vi "水样测试.vi"(11 "数据标记表":string(combo)="N") -> ()   [LabVIEW 2016, in "斯坦道多参数.lvlib"]
panel:
  out "运行状态":u16(ring) items=["空闲", "水样测试", "标样核查"]
  out "多参数运行日志":string
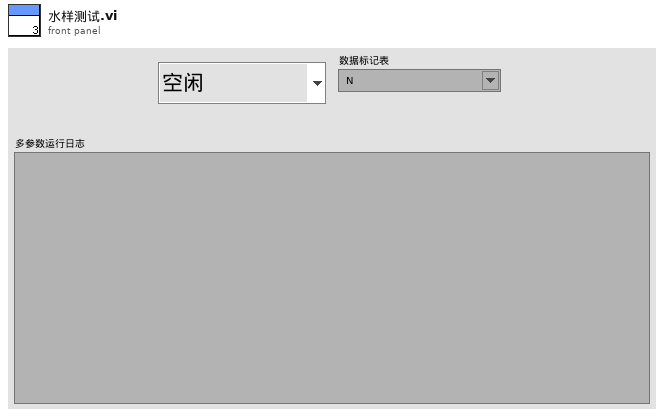
[diagram p1: front panel]
types:
  T1 = cluster{"水样数据时间":timestamp, "水温":dbl, "pH":dbl, "DO":dbl, "DOper":dbl, "电导率":dbl, "ORP":dbl, "浊度":dbl, "叶绿素a":dbl, "藻密度":dbl}
  T2 = cluster{"水温":bool, "pH":bool, "DO":bool, "DOper":bool, "电导率":bool, "ORP":bool, "浊度":bool, "叶绿素a":bool, "藻密度":bool}
  T3 = cluster{"水样数据时间":timestamp, "测量模式":string, "数据类型":string, "水样实测值":sgl, "单位":string, "水样数据标识":string, "信号值":sgl, "标样参考值":sgl, "因子编码":string, "探头温度":sgl}
  T4 = cluster{"ph":bool, "DO":bool, "Cond":bool, "Turb":bool, "叶绿素a":bool, "藻密度":bool, "ORP":bool}
  T5 = cluster{"CH":u16, "监测值":dbl, "温度偏移修正值":sgl, "信号值":sgl}
  T6 = cluster{"温度测量值":sgl, "测量值":sgl, "温度偏移修正值":sgl, "信号值":sgl}
  T7 = cluster{"温度测量值":sgl, "DO%":sgl, "DOmg/L":sgl, "温度偏移修正值":sgl}
  T8 = cluster{"测量量程":dbl, "测量精度":dbl, "测量间隔":dbl, "消解温度":dbl, "消解时长":dbl, "空白校准时间":timestamp, "曲线截距":dbl, "曲线斜率":dbl, "测量检出限":dbl, "测量信号值":dbl, "线性相关系数":dbl, "二次多项式系数":dbl, "标样校准时间":timestamp, "稀释倍数":dbl, "三项式系数":dbl, "空白标定系数":dbl, "量程系数":dbl, "F0/ORPA":dbl, "F1/ORPB":dbl, "F2/ORPK":dbl, "F3":dbl, "F4":dbl, "F5":dbl, "F6":dbl, "F7":dbl, "X0/滴定数":dbl, "量程":dbl}
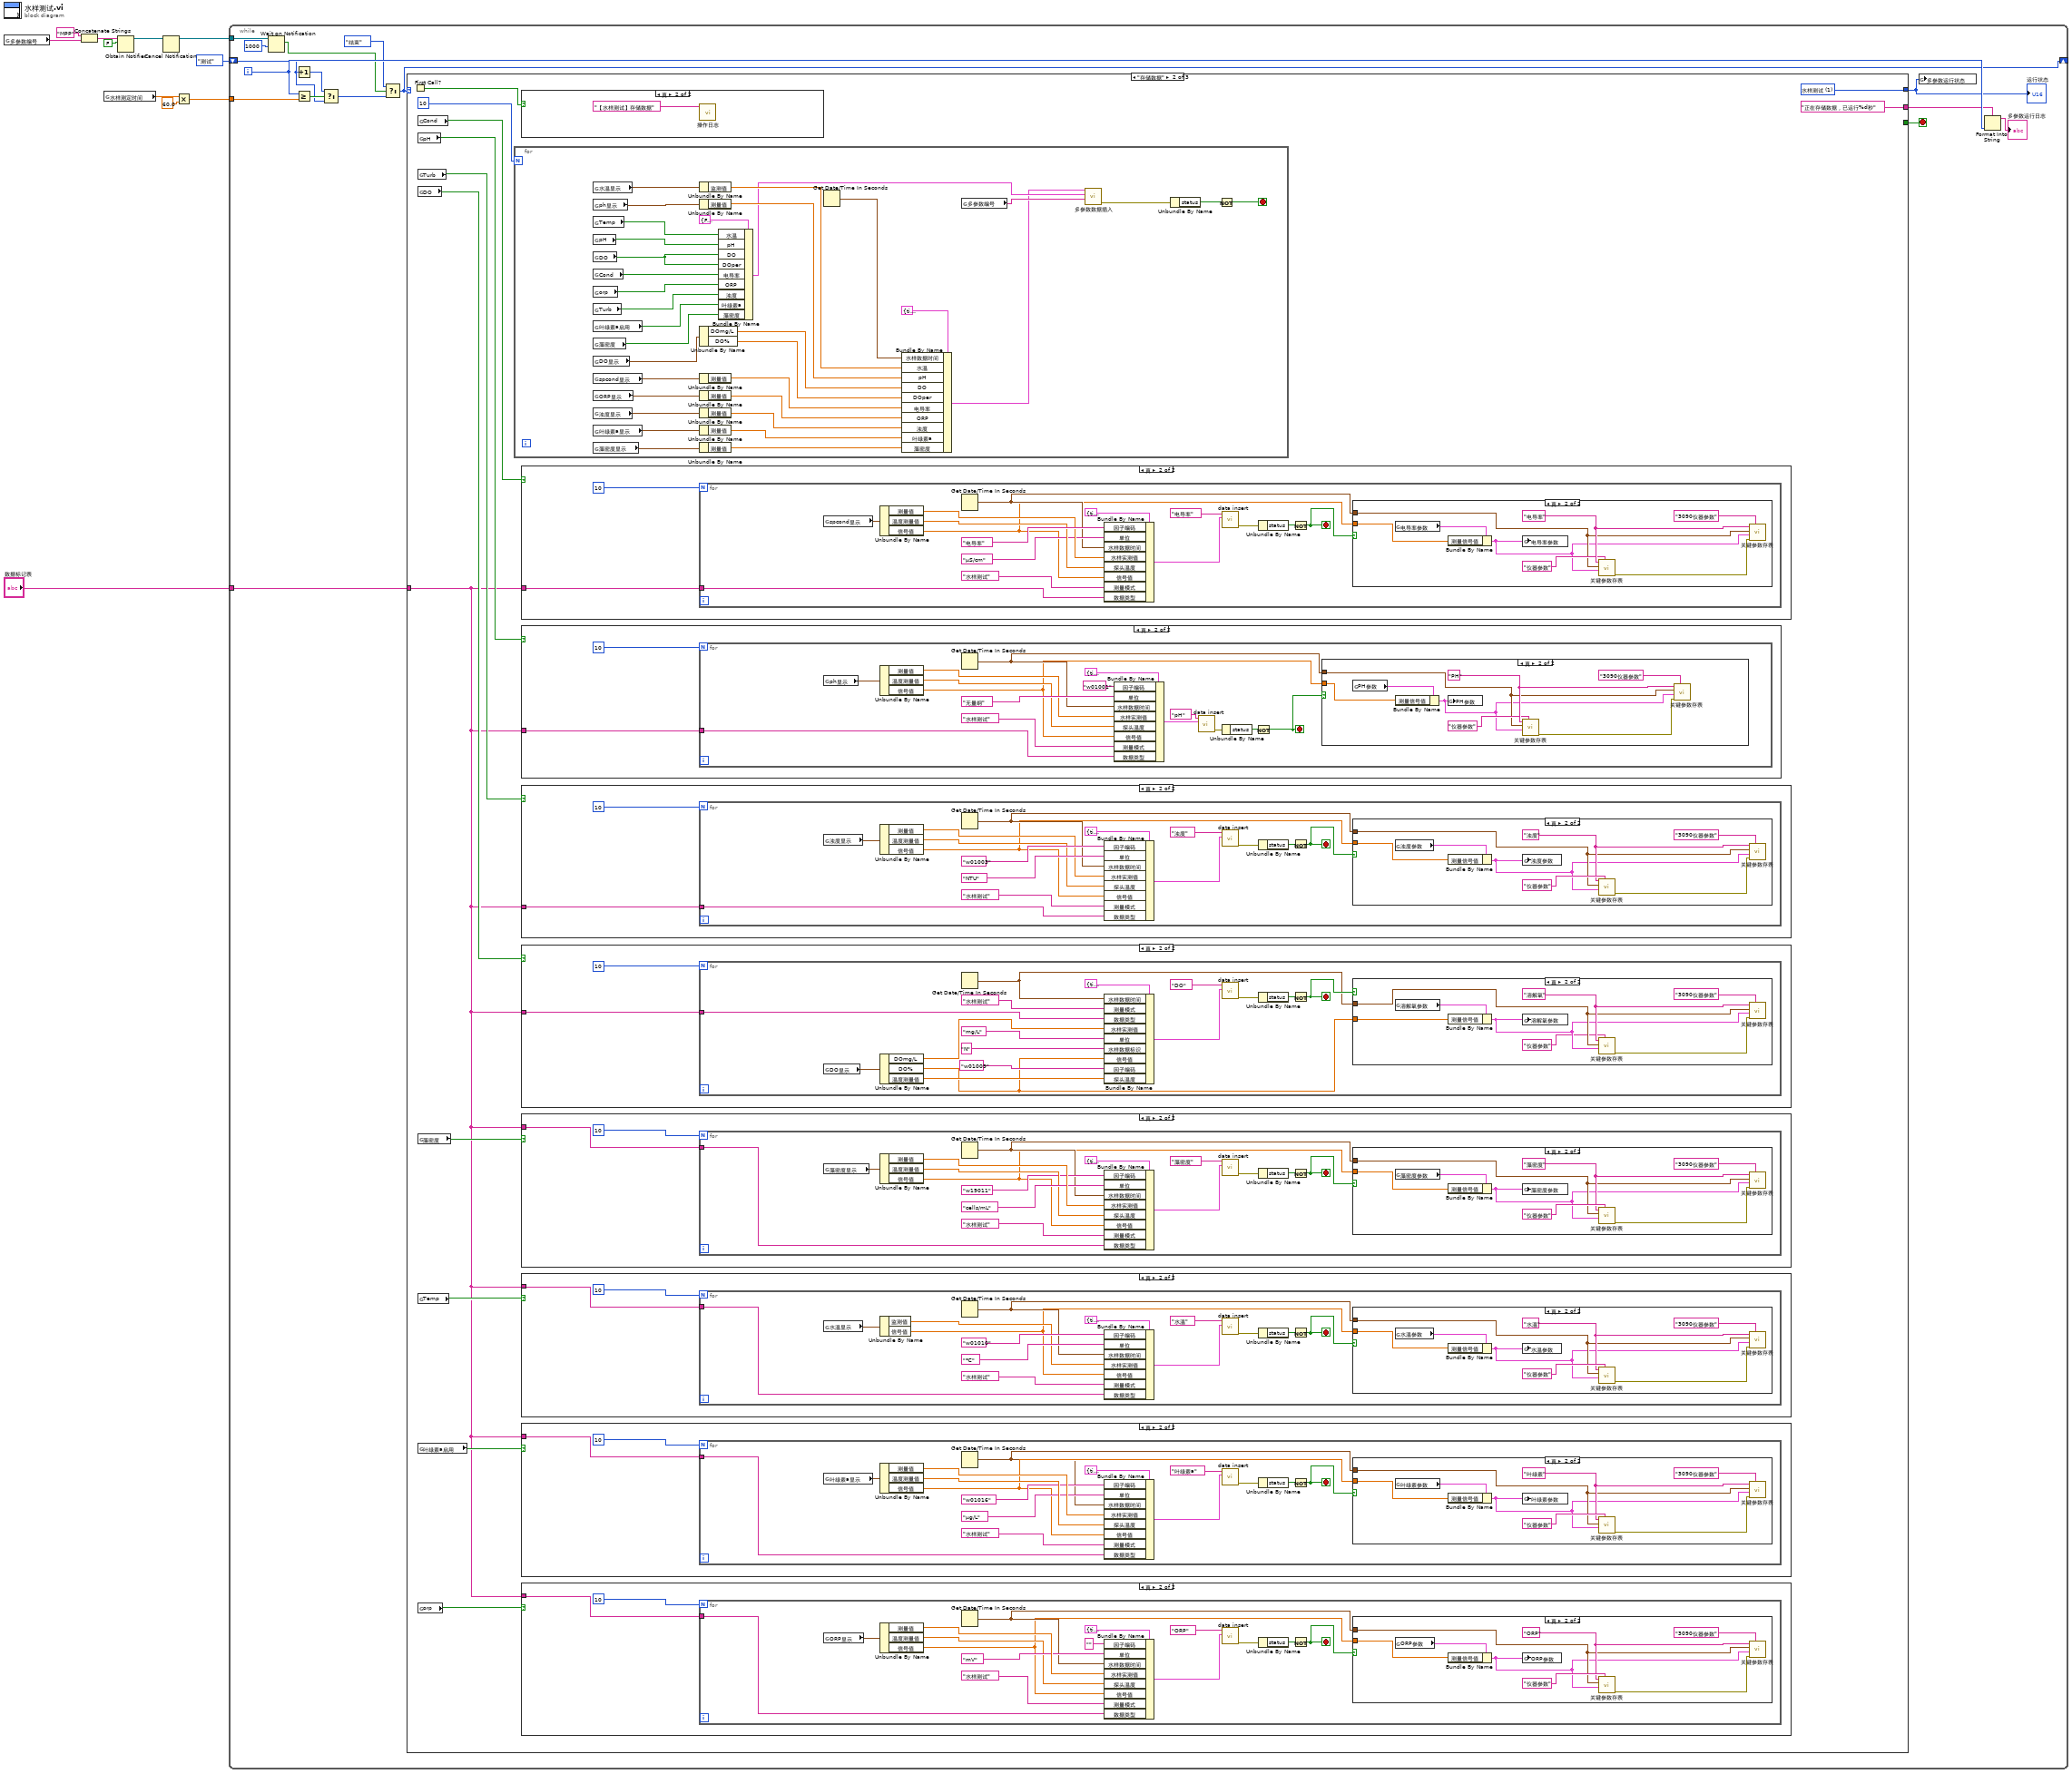
[diagram p0: block diagram]
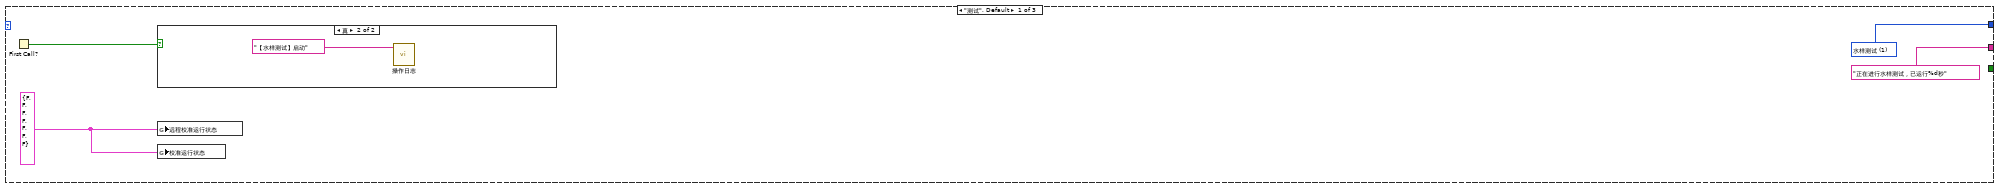
[diagram p2: hidden frame]
diagram:
  n1 = global read "多参数全局变量.vi" "多参数编号"() -> (w2:string)
  n2 = Concatenate Strings("MPP" ("名称（未命名）"), w2) -> (w3:string)
  n3 = global read "断电保存变量.vi" "水样测定时间"() -> (w1:dbl)
  n4 = Obtain Notifier(name (unnamed)=w3, notification data type=FALSE) -> (notifier out=w6:refnum<notifier>)  [unwired: 2 in, 2 out]
  n5 = Cancel Notification(0:w6) -> (8:w5:refnum<notifier>)  [unwired: 1 in, 2 out]
  n6 = Multiply(x=w1, y=60.0) -> (x*y=w10:dbl)
  n7 = while {
    tunnel: w10 -> [w27]
    shift-right: [w14] -> _
    shift-left: enum16{"测试", "存储数据", "结束"}."测试" ("枚举") -> [w21]
    tunnel: w5 -> [w19]
    tunnel: "数据标记表" -> [w13]
    i -> [w25]
    stop <- w26 stop-if-true
    n8 = Wait on Notification(notifier=w19, timeout in ms (-1)=1000 ("超时毫秒(-1)")) -> (notification=w17:bool)  [unwired: 2 in, 3 out]
    n9 = Increment(x=w21) -> (x+1=w20:enum16{"测试", "存储数据", "结束"})
    n10 = Greater Or Equal?(x=w25, y=w27) -> (x >= y?=w22:bool)
    n11 = Select(t=w20, s=w22, f=w21) -> (s? t:f=w15:enum16{"测试", "存储数据", "结束"})
    n12 = Select(t=enum16{"测试", "存储数据", "结束"}."结束" ("枚举"), s=w17, f=w15) -> (s? t:f=w14:enum16{"测试", "存储数据", "结束"})
    n13 = case shown="\"存储数据\"" w14 {
      tunnel: [_ _ TRUE] -> w26
      tunnel: ["正在进行水样测试，已运行%d秒" ("格式字符串") "正在存储数据，已运行%d秒" ("格式字符串") "测试停止，累计运行%d秒" ("格式字符串")] -> w24
      tunnel: [w30 w38 w282] -> w12
      tunnel: w13 -> [_ w35 _]
      frame "测试", Default {
        w28 = T4 {"ph"=FALSE, "DO"=FALSE, "Cond"=FALSE, "Turb"=FALSE, "叶绿素a"=FALSE, "藻密度"=FALSE, "ORP"=FALSE} ("校准运行状态")
        w30 = u16 1 items=["空闲", "水样测试", "标样核查"] ("多参数运行状态")
        n14 = First Call?() -> (First Call?: T/F=w29:bool)
        n15 = case shown="真" w29 {
          frame False {
          }
          frame True {
            n16 = call "操作日志.vi"("日志信息"="【水样测试】启动") -> ()  [unwired: 10 in, 1 out]
          }
        }
        n17 = global write "多参数全局变量.vi" "远程校准运行状态"(w28) -> ()
        n18 = global write "多参数全局变量.vi" "校准运行状态"(w28) -> ()
      }
      frame "存储数据" {
        w38 = u16 1 items=["空闲", "水样测试", "标样核查"] ("多参数运行状态")
        n19 = First Call?() -> (First Call?: T/F=w36:bool)
        n20 = global read "断电保存变量.vi" "Cond"() -> (w43:bool)
        n21 = global read "断电保存变量.vi" "pH"() -> (w41:bool)
        n22 = global read "断电保存变量.vi" "Turb"() -> (w44:bool)
        n23 = global read "断电保存变量.vi" "DO"() -> (w42:bool)
        n24 = global read "断电保存变量.vi" "藻密度"() -> (w37:bool)
        n25 = global read "断电保存变量.vi" "Temp"() -> (w40:bool)
        n26 = global read "断电保存变量.vi" "叶绿素a启用"() -> (w45:bool)
        n27 = global read "断电保存变量.vi" "orp"() -> (w34:bool)
        n28 = for {
          N: 10 -> [_]
          stop <- w49 stop-if-true
          n29 = global read "多参数全局变量.vi" "水温显示"() -> (w78:T5)
          n30 = global read "多参数全局变量.vi" "ph显示"() -> (w76:T6)
          n31 = global read "断电保存变量.vi" "Temp"() -> (w56:bool)
          n32 = global read "断电保存变量.vi" "pH"() -> (w60:bool)
          n33 = global read "断电保存变量.vi" "DO"() -> (w52:bool)
          n34 = global read "断电保存变量.vi" "Cond"() -> (w59:bool)
          n35 = global read "断电保存变量.vi" "orp"() -> (w55:bool)
          n36 = global read "断电保存变量.vi" "Turb"() -> (w58:bool)
          n37 = global read "断电保存变量.vi" "叶绿素a启用"() -> (w54:bool)
          n38 = global read "断电保存变量.vi" "藻密度"() -> (w57:bool)
          n39 = global read "多参数全局变量.vi" "DO显示"() -> (w74:T7)
          n40 = global read "多参数全局变量.vi" "spcond显示"() -> (w71:T6)
          n41 = global read "多参数全局变量.vi" "ORP显示"() -> (w69:T6)
          n42 = global read "多参数全局变量.vi" "浊度显示"() -> (w67:T6)
          n43 = global read "多参数全局变量.vi" "叶绿素a显示"() -> (w63:T6)
          n44 = global read "多参数全局变量.vi" "藻密度显示"() -> (w65:T6)
          n45 = Unbundle By Name(w78) -> ("监测值"=w77:dbl)
          n46 = Unbundle By Name(w76) -> ("测量值"=w75:sgl)
          n47 = Unbundle By Name(w74) -> ("DOmg/L"=w73:sgl, "DO%"=w72:sgl)
          n48 = Unbundle By Name(w71) -> ("测量值"=w70:sgl)
          n49 = Unbundle By Name(w69) -> ("测量值"=w68:sgl)
          n50 = Unbundle By Name(w67) -> ("测量值"=w66:sgl)
          n51 = Unbundle By Name(w63) -> ("测量值"=w62:sgl)
          n52 = Unbundle By Name(w65) -> ("测量值"=w64:sgl)
          n53 = Bundle By Name(cluster=T2 {"水温"=FALSE, "pH"=FALSE, "DO"=FALSE, "DOper"=FALSE, "电导率"=FALSE, "ORP"=FALSE, "浊度"=FALSE, "叶绿素a"=FALSE, "藻密度"=FALSE} ("columns enable"), "水温"=w56, "pH"=w60, "DO"=w52, "DOper"=w52, "电导率"=w59, "ORP"=w55, "浊度"=w58, "叶绿素a"=w54, "藻密度"=w57) -> (w53:T2)
          n54 = Get Date/Time In Seconds() -> (seconds since 1Jan1904=w79:timestamp)
          n55 = Bundle By Name(cluster=T1 {"水样数据时间"=timestamp(0 s since 1904-01-01), "水温"=0.0, "pH"=0.0, "DO"=0.0, "DOper"=0.0, "电导率"=0.0, "ORP"=0.0, "浊度"=0.0, "叶绿素a"=0.0, "藻密度"=0.0} ("data in"), "水样数据时间"=w79, "水温"=w77, "pH"=w75, "DO"=w73, "DOper"=w72, "电导率"=w70, "ORP"=w68, "浊度"=w66, "叶绿素a"=w62, "藻密度"=w64) -> (w46:T1)
          n56 = global read "多参数全局变量.vi" "多参数编号"() -> (w48:string)
          n57 = call "多参数数据插入.vi"("编号"=w48, "columns enable"=w53, "data in"=w46) -> ("error out"=w51:errorcluster)  [unwired: 8 in]
          n58 = Unbundle By Name(w51) -> ("status"=w50:bool)
          n59 = Not(x=w50) -> (.not. x?=w49:bool)
        }
        n60 = case shown="真" w36 {
          frame False {
          }
          frame True {
            n61 = call "操作日志.vi"("日志信息"="【水样测试】存储数据") -> ()  [unwired: 10 in, 1 out]
          }
        }
        n62 = case shown="真" w43 {
          tunnel: w35 -> [_ w182]
          frame False {
          }
          frame True {
            n63 = for {
              N: 10 -> [_]
              tunnel: w182 -> [w183]
              stop <- w189 stop-if-true
              n64 = global read "多参数全局变量.vi" "spcond显示"() -> (w195:T6)
              n65 = Unbundle By Name(w195) -> ("测量值"=w194:sgl, "温度测量值"=w193:sgl, "信号值"=w187:sgl)
              n66 = Get Date/Time In Seconds() -> (seconds since 1Jan1904=w188:timestamp)
              n67 = Bundle By Name(cluster=T3 {"水样数据时间"=timestamp(0 s since 1904-01-01), "测量模式"="", "数据类型"="N", "水样实测值"=0.0, "单位"="", "水样数据标识"="N", "信号值"=0.0, "标样参考值"=0.0, "因子编码"="", "探头温度"=0.0} ("data in"), "因子编码"="电导率", "单位"="μS/cm", "水样数据时间"=w188, "水样实测值"=w194, "探头温度"=w193, "信号值"=w187, "测量模式"="水样测试", "数据类型"=w183) -> (w184:T3)
              n68 = call "data insert.vi"("data in"=w184, "table in"="电导率" ("table输入")) -> ("error out"=w192:errorcluster)  [unwired: 9 in]
              n69 = Unbundle By Name(w192) -> ("status"=w191:bool)
              n70 = Not(x=w191) -> (.not. x?=w189:bool)
              n71 = case shown="真" w189 {
                tunnel: w188 -> [_ w200]
                tunnel: w187 -> [_ w204]
                frame False {
                }
                frame True {
                  w203 = "电导率" ("仪器名称")
                  n72 = global read "断电保存变量.vi" "电导率参数"() -> (w205:T8)
                  n73 = Bundle By Name(cluster=w205, "测量信号值"=w204) -> (w199:T8)
                  n74 = global write "断电保存变量.vi" "电导率参数"(w199) -> ()
                  n75 = call "关键参数存表.vi"("table"="仪器参数", "仪器参数"=w199, "datatime"=w200, "仪器名称"=w203) -> ("error out"=w198:errorcluster)  [unwired: 7 in]
                  n76 = call "关键参数存表.vi"("table"="3090仪器参数", "error in (no error)"=w198, "仪器参数"=w199, "datatime"=w200, "仪器名称"=w203) -> ()  [unwired: 6 in, 1 out]
                }
              }
            }
          }
        }
        n77 = case shown="真" w41 {
          tunnel: w35 -> [_ w233]
          frame False {
          }
          frame True {
            n78 = for {
              N: 10 -> [_]
              tunnel: w233 -> [w234]
              stop <- w239 stop-if-true
              n79 = global read "多参数全局变量.vi" "ph显示"() -> (w244:T6)
              n80 = Unbundle By Name(w244) -> ("测量值"=w243:sgl, "温度测量值"=w242:sgl, "信号值"=w237:sgl)
              n81 = Get Date/Time In Seconds() -> (seconds since 1Jan1904=w238:timestamp)
              n82 = Bundle By Name(cluster=T3 {"水样数据时间"=timestamp(0 s since 1904-01-01), "测量模式"="", "数据类型"="N", "水样实测值"=0.0, "单位"="", "水样数据标识"="N", "信号值"=0.0, "标样参考值"=0.0, "因子编码"="", "探头温度"=0.0} ("data in"), "因子编码"="w01001", "单位"="无量纲", "水样数据时间"=w238, "水样实测值"=w243, "探头温度"=w242, "信号值"=w237, "测量模式"="水样测试", "数据类型"=w234) -> (w248:T3)
              n83 = call "data insert.vi"("data in"=w248, "table in"="pH" ("table输入")) -> ("error out"=w241:errorcluster)  [unwired: 9 in]
              n84 = Unbundle By Name(w241) -> ("status"=w240:bool)
              n85 = Not(x=w240) -> (.not. x?=w239:bool)
              n86 = case shown="真" w239 {
                tunnel: w238 -> [_ w251]
                tunnel: w237 -> [_ w255]
                frame False {
                }
                frame True {
                  w254 = "PH" ("仪器名称")
                  n87 = global read "断电保存变量.vi" "PH参数"() -> (w256:T8)
                  n88 = Bundle By Name(cluster=w256, "测量信号值"=w255) -> (w250:T8)
                  n89 = global write "断电保存变量.vi" "PH参数"(w250) -> ()
                  n90 = call "关键参数存表.vi"("table"="仪器参数", "仪器参数"=w250, "datatime"=w251, "仪器名称"=w254) -> ("error out"=w249:errorcluster)  [unwired: 7 in]
                  n91 = call "关键参数存表.vi"("table"="3090仪器参数", "error in (no error)"=w249, "仪器参数"=w250, "datatime"=w251, "仪器名称"=w254) -> ()  [unwired: 6 in, 1 out]
                }
              }
            }
          }
        }
        n92 = case shown="真" w44 {
          tunnel: w35 -> [_ w157]
          frame False {
          }
          frame True {
            n93 = for {
              N: 10 -> [_]
              tunnel: w157 -> [w158]
              stop <- w163 stop-if-true
              n94 = global read "多参数全局变量.vi" "浊度显示"() -> (w168:T6)
              n95 = Unbundle By Name(w168) -> ("测量值"=w167:sgl, "温度测量值"=w166:sgl, "信号值"=w161:sgl)
              n96 = Get Date/Time In Seconds() -> (seconds since 1Jan1904=w162:timestamp)
              n97 = Bundle By Name(cluster=T3 {"水样数据时间"=timestamp(0 s since 1904-01-01), "测量模式"="", "数据类型"="N", "水样实测值"=0.0, "单位"="", "水样数据标识"="N", "信号值"=0.0, "标样参考值"=0.0, "因子编码"="", "探头温度"=0.0} ("data in"), "因子编码"="w01003", "单位"="NTU", "水样数据时间"=w162, "水样实测值"=w167, "探头温度"=w166, "信号值"=w161, "测量模式"="水样测试", "数据类型"=w158) -> (w171:T3)
              n98 = call "data insert.vi"("data in"=w171, "table in"="浊度" ("table输入")) -> ("error out"=w165:errorcluster)  [unwired: 9 in]
              n99 = Unbundle By Name(w165) -> ("status"=w164:bool)
              n100 = Not(x=w164) -> (.not. x?=w163:bool)
              n101 = case shown="真" w163 {
                tunnel: w162 -> [_ w175]
                tunnel: w161 -> [_ w179]
                frame False {
                }
                frame True {
                  w176 = "浊度" ("仪器名称")
                  n102 = global read "断电保存变量.vi" "浊度参数"() -> (w180:T8)
                  n103 = Bundle By Name(cluster=w180, "测量信号值"=w179) -> (w174:T8)
                  n104 = global write "断电保存变量.vi" "浊度参数"(w174) -> ()
                  n105 = call "关键参数存表.vi"("table"="仪器参数", "仪器参数"=w174, "datatime"=w175, "仪器名称"=w176) -> ("error out"=w173:errorcluster)  [unwired: 7 in]
                  n106 = call "关键参数存表.vi"("table"="3090仪器参数", "error in (no error)"=w173, "仪器参数"=w174, "datatime"=w175, "仪器名称"=w176) -> ()  [unwired: 6 in, 1 out]
                }
              }
            }
          }
        }
        n107 = case shown="真" w42 {
          tunnel: w35 -> [_ w207]
          frame False {
          }
          frame True {
            n108 = for {
              N: 10 -> [_]
              tunnel: w207 -> [w218]
              stop <- w222 stop-if-true
              n109 = global read "多参数全局变量.vi" "DO显示"() -> (w223:T7)
              n110 = Unbundle By Name(w223) -> ("DOmg/L"=w217:sgl, "DO%"=w210:sgl, "温度测量值"=w211:sgl)
              n111 = Get Date/Time In Seconds() -> (seconds since 1Jan1904=w220:timestamp)
              n112 = Bundle By Name(cluster=T3 {"水样数据时间"=timestamp(0 s since 1904-01-01), "测量模式"="", "数据类型"="N", "水样实测值"=0.0, "单位"="", "水样数据标识"="N", "信号值"=0.0, "标样参考值"=0.0, "因子编码"="", "探头温度"=0.0} ("data in"), "水样数据时间"=w220, "测量模式"="水样测试", "数据类型"=w218, "水样实测值"=w217, "单位"="mg/L", "水样数据标识"="N", "信号值"=w210, "因子编码"="w01009", "探头温度"=w211) -> (w208:T3)
              n113 = call "data insert.vi"("data in"=w208, "table in"="DO") -> ("error out"=w213:errorcluster)  [unwired: 9 in]
              n114 = Unbundle By Name(w213) -> ("status"=w214:bool)
              n115 = Not(x=w214) -> (.not. x?=w222:bool)
              n116 = case shown="真" w222 {
                tunnel: w220 -> [_ w228]
                tunnel: w210 -> [_ w230]
                frame False {
                }
                frame True {
                  w229 = "溶解氧" ("仪器名称")
                  n117 = global read "断电保存变量.vi" "溶解氧参数"() -> (w231:T8)
                  n118 = Bundle By Name(cluster=w231, "测量信号值"=w230) -> (w227:T8)
                  n119 = global write "断电保存变量.vi" "溶解氧参数"(w227) -> ()
                  n120 = call "关键参数存表.vi"("table"="仪器参数", "仪器参数"=w227, "datatime"=w228, "仪器名称"=w229) -> ("error out"=w226:errorcluster)  [unwired: 7 in]
                  n121 = call "关键参数存表.vi"("table"="3090仪器参数", "error in (no error)"=w226, "仪器参数"=w227, "datatime"=w228, "仪器名称"=w229) -> ()  [unwired: 6 in, 1 out]
                }
              }
            }
          }
        }
        n122 = case shown="真" w37 {
          tunnel: w35 -> [_ w107]
          frame False {
          }
          frame True {
            n123 = for {
              N: 10 -> [_]
              tunnel: w107 -> [w109]
              stop <- w111 stop-if-true
              n124 = global read "多参数全局变量.vi" "藻密度显示"() -> (w117:T6)
              n125 = Unbundle By Name(w117) -> ("测量值"=w122:sgl, "温度测量值"=w120:sgl, "信号值"=w112:sgl)
              n126 = Get Date/Time In Seconds() -> (seconds since 1Jan1904=w113:timestamp)
              n127 = Bundle By Name(cluster=T3 {"水样数据时间"=timestamp(0 s since 1904-01-01), "测量模式"="", "数据类型"="N", "水样实测值"=0.0, "单位"="", "水样数据标识"="N", "信号值"=0.0, "标样参考值"=0.0, "因子编码"="", "探头温度"=0.0} ("data in"), "因子编码"="w19011", "单位"="cells/mL", "水样数据时间"=w113, "水样实测值"=w122, "探头温度"=w120, "信号值"=w112, "测量模式"="水样测试", "数据类型"=w109) -> (w114:T3)
              n128 = call "data insert.vi"("data in"=w114, "table in"="藻密度" ("table输入")) -> ("error out"=w116:errorcluster)  [unwired: 9 in]
              n129 = Unbundle By Name(w116) -> ("status"=w115:bool)
              n130 = Not(x=w115) -> (.not. x?=w111:bool)
              n131 = case shown="真" w111 {
                tunnel: w113 -> [_ w126]
                tunnel: w112 -> [_ w129]
                frame False {
                }
                frame True {
                  w127 = "藻密度" ("仪器名称")
                  n132 = global read "断电保存变量.vi" "藻密度参数"() -> (w130:T8)
                  n133 = Bundle By Name(cluster=w130, "测量信号值"=w129) -> (w125:T8)
                  n134 = global write "断电保存变量.vi" "藻密度参数"(w125) -> ()
                  n135 = call "关键参数存表.vi"("table"="仪器参数", "仪器参数"=w125, "datatime"=w126, "仪器名称"=w127) -> ("error out"=w124:errorcluster)  [unwired: 7 in]
                  n136 = call "关键参数存表.vi"("table"="3090仪器参数", "error in (no error)"=w124, "仪器参数"=w125, "datatime"=w126, "仪器名称"=w127) -> ()  [unwired: 6 in, 1 out]
                }
              }
            }
          }
        }
        n137 = case shown="真" w40 {
          tunnel: w35 -> [_ w258]
          frame False {
          }
          frame True {
            n138 = for {
              N: 10 -> [_]
              tunnel: w258 -> [w259]
              stop <- w264 stop-if-true
              n139 = global read "多参数全局变量.vi" "水温显示"() -> (w268:T5)
              n140 = Unbundle By Name(w268) -> ("监测值"=w267:dbl, "信号值"=w262:sgl)
              n141 = Get Date/Time In Seconds() -> (seconds since 1Jan1904=w263:timestamp)
              n142 = Bundle By Name(cluster=T3 {"水样数据时间"=timestamp(0 s since 1904-01-01), "测量模式"="", "数据类型"="N", "水样实测值"=0.0, "单位"="", "水样数据标识"="N", "信号值"=0.0, "标样参考值"=0.0, "因子编码"="", "探头温度"=0.0} ("data in"), "因子编码"="w01010", "单位"="℃", "水样数据时间"=w263, "水样实测值"=w267, "信号值"=w262, "测量模式"="水样测试", "数据类型"=w259) -> (w271:T3)
              n143 = call "data insert.vi"("data in"=w271, "table in"="水温" ("table输入")) -> ("error out"=w266:errorcluster)  [unwired: 9 in]
              n144 = Unbundle By Name(w266) -> ("status"=w265:bool)
              n145 = Not(x=w265) -> (.not. x?=w264:bool)
              n146 = case shown="真" w264 {
                tunnel: w263 -> [_ w276]
                tunnel: w262 -> [_ w279]
                frame False {
                }
                frame True {
                  w277 = "水温" ("仪器名称")
                  n147 = global read "断电保存变量.vi" "水温参数"() -> (w280:T8)
                  n148 = Bundle By Name(cluster=w280, "测量信号值"=w279) -> (w275:T8)
                  n149 = global write "断电保存变量.vi" "水温参数"(w275) -> ()
                  n150 = call "关键参数存表.vi"("table"="仪器参数", "仪器参数"=w275, "datatime"=w276, "仪器名称"=w277) -> ("error out"=w274:errorcluster)  [unwired: 7 in]
                  n151 = call "关键参数存表.vi"("table"="3090仪器参数", "error in (no error)"=w274, "仪器参数"=w275, "datatime"=w276, "仪器名称"=w277) -> ()  [unwired: 6 in, 1 out]
                }
              }
            }
          }
        }
        n152 = case shown="真" w45 {
          tunnel: w35 -> [_ w132]
          frame False {
          }
          frame True {
            n153 = for {
              N: 10 -> [_]
              tunnel: w132 -> [w133]
              stop <- w138 stop-if-true
              n154 = global read "多参数全局变量.vi" "叶绿素a显示"() -> (w142:T6)
              n155 = Unbundle By Name(w142) -> ("测量值"=w147:sgl, "温度测量值"=w146:sgl, "信号值"=w137:sgl)
              n156 = Get Date/Time In Seconds() -> (seconds since 1Jan1904=w136:timestamp)
              n157 = Bundle By Name(cluster=T3 {"水样数据时间"=timestamp(0 s since 1904-01-01), "测量模式"="", "数据类型"="N", "水样实测值"=0.0, "单位"="", "水样数据标识"="N", "信号值"=0.0, "标样参考值"=0.0, "因子编码"="", "探头温度"=0.0} ("data in"), "因子编码"="w01016", "单位"="μg/L", "水样数据时间"=w136, "水样实测值"=w147, "探头温度"=w146, "信号值"=w137, "测量模式"="水样测试", "数据类型"=w133) -> (w144:T3)
              n158 = call "data insert.vi"("data in"=w144, "table in"="叶绿素a" ("table输入")) -> ("error out"=w141:errorcluster)  [unwired: 9 in]
              n159 = Unbundle By Name(w141) -> ("status"=w140:bool)
              n160 = Not(x=w140) -> (.not. x?=w138:bool)
              n161 = case shown="真" w138 {
                tunnel: w136 -> [_ w150]
                tunnel: w137 -> [_ w154]
                frame False {
                }
                frame True {
                  w151 = "叶绿素" ("仪器名称")
                  n162 = global read "断电保存变量.vi" "叶绿素参数"() -> (w155:T8)
                  n163 = Bundle By Name(cluster=w155, "测量信号值"=w154) -> (w149:T8)
                  n164 = global write "断电保存变量.vi" "叶绿素参数"(w149) -> ()
                  n165 = call "关键参数存表.vi"("table"="仪器参数", "仪器参数"=w149, "datatime"=w150, "仪器名称"=w151) -> ("error out"=w148:errorcluster)  [unwired: 7 in]
                  n166 = call "关键参数存表.vi"("table"="3090仪器参数", "error in (no error)"=w148, "仪器参数"=w149, "datatime"=w150, "仪器名称"=w151) -> ()  [unwired: 6 in, 1 out]
                }
              }
            }
          }
        }
        n167 = case shown="真" w34 {
          tunnel: w35 -> [_ w81]
          frame False {
          }
          frame True {
            n168 = for {
              N: 10 -> [_]
              tunnel: w81 -> [w83]
              stop <- w88 stop-if-true
              n169 = global read "多参数全局变量.vi" "ORP显示"() -> (w92:T6)
              n170 = Unbundle By Name(w92) -> ("测量值"=w96:sgl, "温度测量值"=w94:sgl, "信号值"=w86:sgl)
              n171 = Get Date/Time In Seconds() -> (seconds since 1Jan1904=w87:timestamp)
              n172 = Bundle By Name(cluster=T3 {"水样数据时间"=timestamp(0 s since 1904-01-01), "测量模式"="", "数据类型"="N", "水样实测值"=0.0, "单位"="", "水样数据标识"="N", "信号值"=0.0, "标样参考值"=0.0, "因子编码"="", "探头温度"=0.0} ("data in"), "因子编码"="", "单位"="mV", "水样数据时间"=w87, "水样实测值"=w96, "探头温度"=w94, "信号值"=w86, "测量模式"="水样测试", "数据类型"=w83) -> (w84:T3)
              n173 = call "data insert.vi"("data in"=w84, "table in"="ORP" ("table输入")) -> ("error out"=w91:errorcluster)  [unwired: 9 in]
              n174 = Unbundle By Name(w91) -> ("status"=w90:bool)
              n175 = Not(x=w90) -> (.not. x?=w88:bool)
              n176 = case shown="真" w88 {
                tunnel: w87 -> [_ w100]
                tunnel: w86 -> [_ w103]
                frame False {
                }
                frame True {
                  w101 = "ORP" ("仪器名称")
                  n177 = global read "断电保存变量.vi" "ORP参数"() -> (w104:T8)
                  n178 = Bundle By Name(cluster=w104, "测量信号值"=w103) -> (w99:T8)
                  n179 = global write "断电保存变量.vi" "ORP参数"(w99) -> ()
                  n180 = call "关键参数存表.vi"("table"="仪器参数", "仪器参数"=w99, "datatime"=w100, "仪器名称"=w101) -> ("error out"=w98:errorcluster)  [unwired: 7 in]
                  n181 = call "关键参数存表.vi"("table"="3090仪器参数", "error in (no error)"=w98, "仪器参数"=w99, "datatime"=w100, "仪器名称"=w101) -> ()  [unwired: 6 in, 1 out]
                }
              }
            }
          }
        }
      }
      frame "结束" {
        w282 = u16 0 items=["空闲", "水样测试", "标样核查"] ("多参数运行状态")
        n182 = First Call?() -> (First Call?: T/F=w281:bool)
        n183 = case shown="真" w281 {
          frame False {
          }
          frame True {
            n184 = call "操作日志.vi"("日志信息"="【水样测试】结束") -> ()  [unwired: 10 in, 1 out]
          }
        }
      }
    }
    "运行状态" <- w12
    n185 = global write "多参数全局变量.vi" "多参数运行状态"(w12) -> ()
    n186 = Format Into String(format string=w24, w25) -> (resulting string=→"多参数运行日志":string)  [unwired: 2 in, 1 out]
  }
